vi "lvstyx_read_all_path_bool.vi"(7 "Log? (T)":bool=TRUE, 8 "error in (no error)":errorcluster, 10 "path":string, 11 "client ptr":u32) -> (0 "error out":errorcluster, 2 "bool":bool, 3 "dup client ptr":u32)   [LabVIEW 2010, in "lib1299.lvlib"]
uses:
  lib1299.lvlib
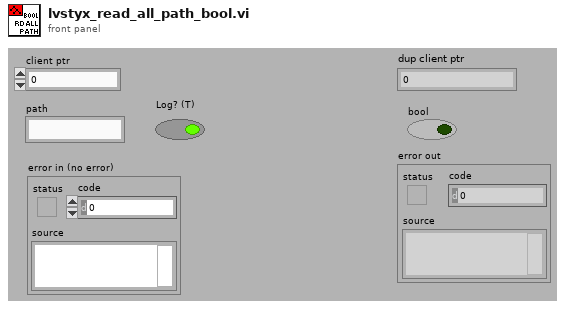
[diagram p1: front panel]
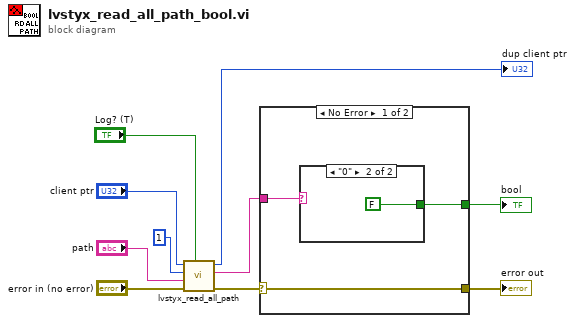
[diagram p0: block diagram]
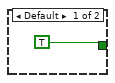
[diagram p2: hidden frame]
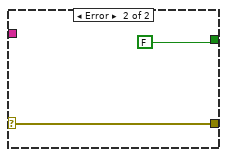
[diagram p3: hidden frame]
diagram:
  n1 = call "lvstyx_read_all_path.vi"("Log? (T)"="Log? (T)", "error in (no error)"="error in (no error)", "path"="path", "lim"=1, "client ptr"="client ptr") -> ("error out"=w10:errorcluster, "buf"=w9:string, "dup client ptr"=→"dup client ptr":u32)  [unwired: 4 in]
  n2 = case shown="No Error" w10 {
    selector: w10 -> [w13 w17]
    tunnel: w9 -> [w12 _]
    tunnel: [w13 w17] -> w6
    tunnel: [w11 FALSE] -> w2
    frame No Error {
      n3 = case shown="\"0\"" w12 {
        tunnel: [TRUE FALSE] -> w11
        frame Default {
        }
        frame "0" {
        }
      }
    }
    frame Error {
    }
  }
  "error out" <- w6
  "bool" <- w2
